vi "智慧外卖登录.vi"() -> ()   [LabVIEW 2020]
panel:
  in  "退出":bool
  in  "登录类型：":string(combo)="普通用户"
  in  "密      码：":string
  in  "用      户：":string
  in  "修改密码":bool
  in  "注册":bool
  in  "登录":bool
  out "登录状态":bool
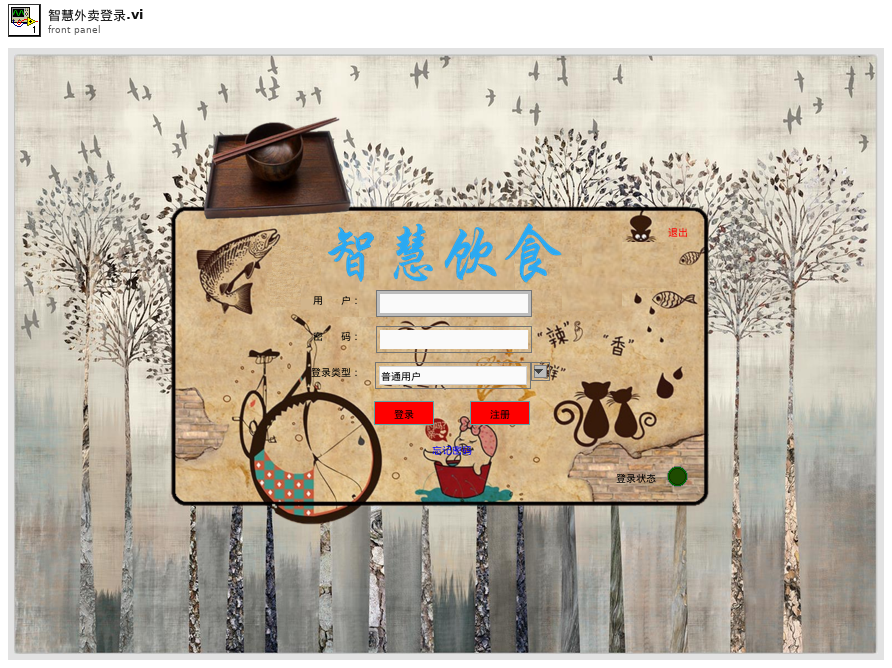
[diagram p1: front panel]
types:
  T1 = typedef "Sound Output Task ID.ctl" = u32
  T2 = enum32{"Invalid", "Standard", "Closed", "Hidden", "Minimized", "Maximized"}
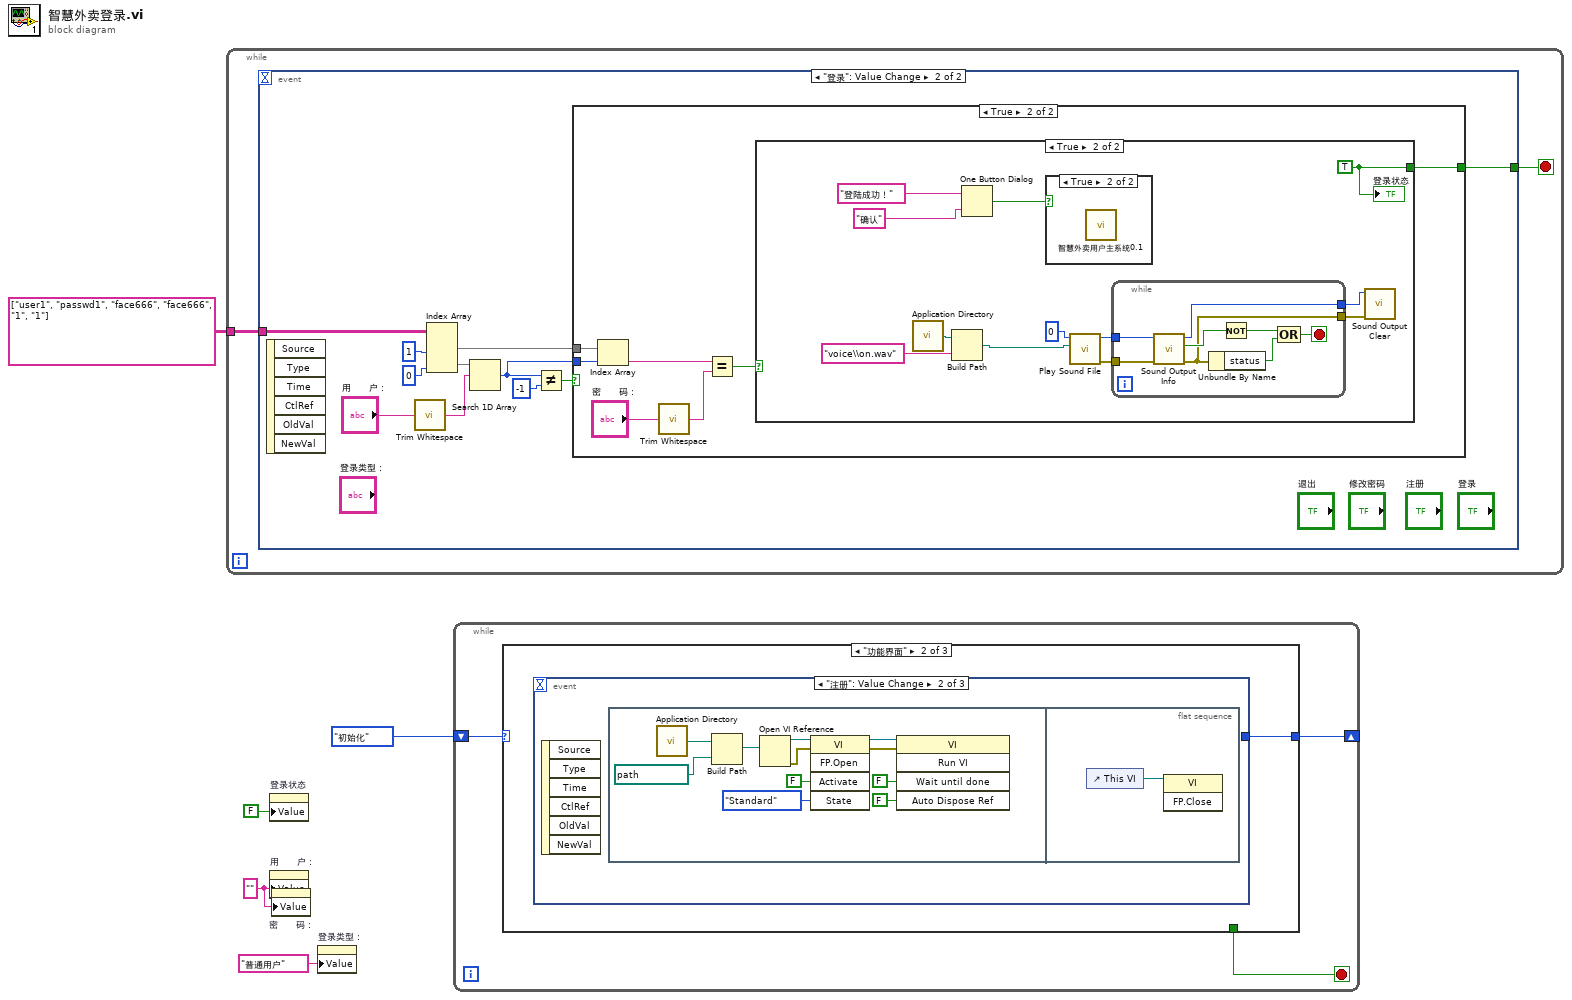
[diagram p0: block diagram]
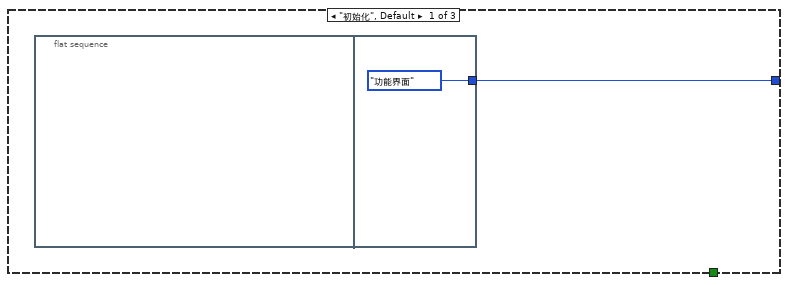
[diagram p2: hidden frame]
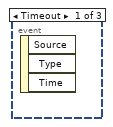
[diagram p3: hidden frame]
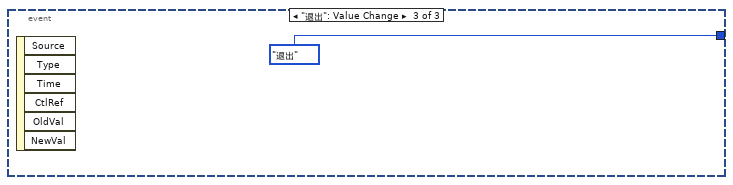
[diagram p4: hidden frame]
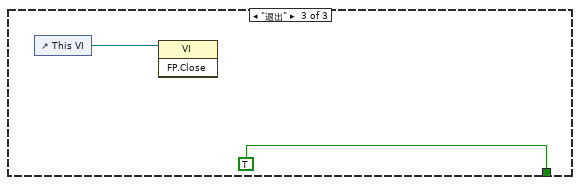
[diagram p5: hidden frame]
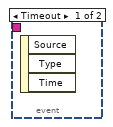
[diagram p6: hidden frame]
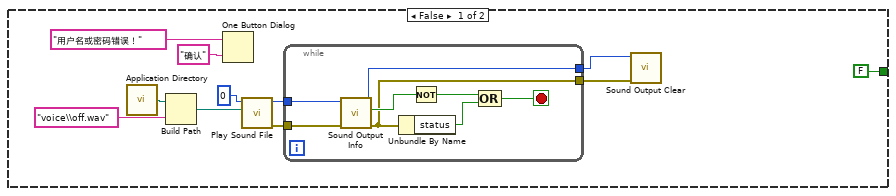
[diagram p7: hidden frame]
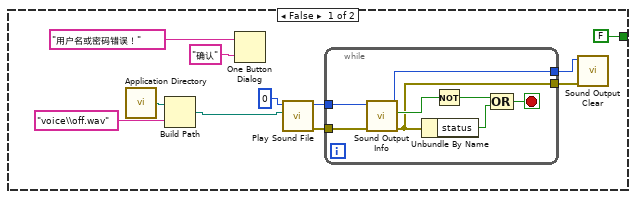
[diagram p8: hidden frame]
diagram:
  w2 = "" ("用户名：")
  n1 = while {
    tunnel: string[][] [["user1", "passwd1"], ["face666", "face666"], ["1", "1"]] -> [w7]
    stop <- w6 stop-if-true
    n2 = event shown="[1] \"登录\": Value Change" {
      selector: _ -> [_ _]
      dyn-events: _ -> [_ _]
      timeout: _ -> [_ _]
      tunnel: w7 -> [_ w18]
      tunnel: [_ w10] -> w6
      event Timeout {
        n3 = event-data() -> ()  [unwired: 1 in, 3 out]
      }
      event "登录": Value Change {
        n4 = event-data() -> ()  [unwired: 1 in, 6 out]
        n5 = call <vilib>:"Trim Whitespace.vi"("string"="用      户：") -> ("trimmed string"=w8:string)  [unwired: 1 in]
        n6 = Index Array(array=w18, index (col) #1=1 ("禁用的索引 (列)"), index (col) #2=0 ("索引 (列)")) -> (element #1=w13:string[], element #2=w15:string[])  [unwired: 2 in]
        n7 = Search 1D Array(1D array=w15, element=w8) -> (index of element=w12:i32)  [unwired: 1 in]
        n8 = Not Equal?(x=w12, y=-1) -> (x != y?=w11:bool)
        n9 = case shown="True" w11 {
          tunnel: w13 -> [_ w44]
          tunnel: w12 -> [_ w43]
          tunnel: [FALSE w40] -> w10
          frame False {
            n10 = call <vilib>:"Application Directory.vi"() -> ("Application Directory"=w21:path)
            n11 = Build Path(base path=w21, name or relative path="voice\\off.wav" ("名称或相对路径")) -> (appended path=w26:path)
            n12 = One Button Dialog(message="用户名或密码错误！" ("消息"), button name ("OK")="确认" ("按钮名称（“确定”）")) -> ()  [unwired: 1 out]
            n13 = call <vilib>:"Play Sound File.vi"("path"=w26, "device ID"=u32 0) -> ("error out"=w22:errorcluster, "task ID"=w23:T1)  [unwired: 8 in]
            n14 = while {
              tunnel: w22 -> [w37]
              tunnel: w23 -> [w36]
              tunnel: [w31] -> w24
              tunnel: [w30] -> w25
              stop <- w33 stop-if-true
              n15 = call <vilib>:"Sound Output Info.vi"("error in (no error)"=w37, "task ID"=w36) -> ("error out"=w30:errorcluster, "is playing?"=w35:bool, "task ID out"=w31:T1)  [unwired: 6 in, 1 out]
              n16 = Unbundle By Name(w30) -> ("status"=w32:bool)
              n17 = Not(x=w35) -> (.not. x?=w34:bool)
              n18 = Compound Arithmetic op=OR(w34, w32) -> (w33:bool)
            }
            n19 = call <vilib>:"Sound Output Clear.vi"("error in (no error)"=w25, "task ID"=w24) -> ()  [unwired: 9 in, 1 out]
          }
          frame True {
            n20 = Index Array(array=w44, index=w43) -> (element=w42:string)
            n21 = call <vilib>:"Trim Whitespace.vi"("string"="密      码：") -> ("trimmed string"=w38:string)  [unwired: 1 in]
            n22 = Equal?(x=w42, y=w38) -> (x = y?=w41:bool)
            n23 = case shown="True" w41 {
              tunnel: [FALSE w75] -> w40
              frame False {
                n24 = call <vilib>:"Application Directory.vi"() -> ("Application Directory"=w49:path)
                n25 = Build Path(base path=w49, name or relative path="voice\\off.wav" ("名称或相对路径")) -> (appended path=w54:path)
                n26 = One Button Dialog(message="用户名或密码错误！" ("消息"), button name ("OK")="确认" ("按钮名称（“确定”）")) -> ()  [unwired: 1 out]
                n27 = call <vilib>:"Play Sound File.vi"("path"=w54, "device ID"=u32 0) -> ("error out"=w50:errorcluster, "task ID"=w51:T1)  [unwired: 8 in]
                n28 = while {
                  tunnel: w50 -> [w63]
                  tunnel: w51 -> [w62]
                  tunnel: [w57] -> w52
                  tunnel: [w56] -> w53
                  stop <- w59 stop-if-true
                  n29 = call <vilib>:"Sound Output Info.vi"("error in (no error)"=w63, "task ID"=w62) -> ("error out"=w56:errorcluster, "is playing?"=w61:bool, "task ID out"=w57:T1)  [unwired: 6 in, 1 out]
                  n30 = Unbundle By Name(w56) -> ("status"=w58:bool)
                  n31 = Not(x=w61) -> (.not. x?=w60:bool)
                  n32 = Compound Arithmetic op=OR(w60, w58) -> (w59:bool)
                }
                n33 = call <vilib>:"Sound Output Clear.vi"("error in (no error)"=w53, "task ID"=w52) -> ()  [unwired: 9 in, 1 out]
              }
              frame True {
                w75 = TRUE
                n34 = call <vilib>:"Application Directory.vi"() -> ("Application Directory"=w64:path)
                n35 = Build Path(base path=w64, name or relative path="voice\\on.wav" ("名称或相对路径")) -> (appended path=w71:path)
                n36 = One Button Dialog(message="登陆成功！" ("消息"), button name ("OK")="确认" ("按钮名称（“确定”）")) -> (true=w72:bool)
                n37 = case shown="True" w72 {
                  frame False {
                  }
                  frame True {
                    n38 = call "智慧外卖用户主系统0.1.vi"() -> ()  [unwired: 12 in]
                  }
                }
                n39 = call <vilib>:"Play Sound File.vi"("path"=w71, "device ID"=u32 0) -> ("error out"=w67:errorcluster, "task ID"=w68:T1)  [unwired: 8 in]
                n40 = while {
                  tunnel: w67 -> [w83]
                  tunnel: w68 -> [w82]
                  tunnel: [w77] -> w69
                  tunnel: [w76] -> w70
                  stop <- w79 stop-if-true
                  n41 = call <vilib>:"Sound Output Info.vi"("error in (no error)"=w83, "task ID"=w82) -> ("error out"=w76:errorcluster, "is playing?"=w81:bool, "task ID out"=w77:T1)  [unwired: 6 in, 1 out]
                  n42 = Unbundle By Name(w76) -> ("status"=w78:bool)
                  n43 = Not(x=w81) -> (.not. x?=w80:bool)
                  n44 = Compound Arithmetic op=OR(w80, w78) -> (w79:bool)
                }
                n45 = call <vilib>:"Sound Output Clear.vi"("error in (no error)"=w70, "task ID"=w69) -> ()  [unwired: 9 in, 1 out]
                "登录状态" <- w75
              }
            }
          }
        }
      }
    }
  }
  n46 = property on="登录状态" class="Bool (strict)"("Value"=FALSE) -> ()  [unwired: 2 in, 2 out]
  n47 = property on="用      户：" class="Str"("Value"=w2) -> ()  [unwired: 2 in, 2 out]
  n48 = property on="密      码：" class="Str"("Value"=w2) -> ()  [unwired: 2 in, 2 out]
  n49 = property on="登录类型：" class="CmbBox"("Value"="普通用户" ("登录类型：")) -> ()  [unwired: 2 in, 2 out]
  n50 = while {
    shift-right: [w85] -> _
    shift-left: enum16{"初始化", "功能界面", "退出"}."初始化" ("功能") -> [w86]
    stop <- w84 stop-if-true
    n51 = case shown="\"功能界面\"" w86 {
      tunnel: [w87 w89 _] -> w85
      tunnel: [_ _ TRUE] -> w84
      frame "初始化", Default {
        n52 = flat-sequence {
          tunnel: [enum16{"初始化", "功能界面", "退出"}."功能界面" ("功能")] -> w87
          frame #0 {
          }
          frame #1 {
          }
        }
      }
      frame "功能界面" {
        n53 = event shown="[1] \"注册\": Value Change" {
          selector: _ -> [_ _ _]
          dyn-events: _ -> [_ _ _]
          timeout: _ -> [_ _ _]
          tunnel: [_ _ enum16{"初始化", "功能界面", "退出"}."退出" ("功能")] -> w89
          event Timeout {
            n54 = event-data() -> ()  [unwired: 1 in, 3 out]
          }
          event "注册": Value Change {
            n55 = event-data() -> ()  [unwired: 1 in, 6 out]
            n56 = flat-sequence {
              frame #0 {
                n57 = call <vilib>:"Application Directory.vi"() -> ("Application Directory"=w100:path)
                n58 = Build Path(base path=w100, name or relative path=path "用户注册.vi") -> (appended path=w98:path)
                n59 = Open VI Reference(vi path=w98) -> (vi reference=w97:refnum<vi>, error out=w96:errorcluster)  [unwired: 5 in]
                n60 = invoke class="VI" method="FP.Open"(reference=w97, error in=w96, "Activate"=FALSE ("Activate?"), "State"=T2."Standard") -> (reference out=w93:refnum<vi>, error out=w92:errorcluster)  [unwired: 1 in, 3 out]
                n61 = invoke class="VI" method="Run VI"(reference=w93, error in=w92, "Wait until done"=FALSE ("Wait Until Done"), "Auto Dispose Ref"=FALSE ("Auto Dispose Reference")) -> ()  [unwired: 1 in, 5 out]
              }
              frame #1 {
                n62 = control-ref of="This VI"() -> (w101:refnum<vi>)
                n63 = invoke class="VI" method="FP.Close"(reference=w101) -> ()  [unwired: 2 in, 3 out]
              }
            }
          }
          event "退出": Value Change {
            n64 = event-data() -> ()  [unwired: 1 in, 6 out]
          }
        }
      }
      frame "退出" {
        n65 = control-ref of="This VI"() -> (w103:refnum<vi>)
        n66 = invoke class="VI" method="FP.Close"(reference=w103) -> ()  [unwired: 2 in, 3 out]
      }
    }
  }
